vi "Main Chroma 19053 hipot.vi"   [LabVIEW 2018]
types:
  T1 = cluster{"error":bool, "code":i8, "source":string}
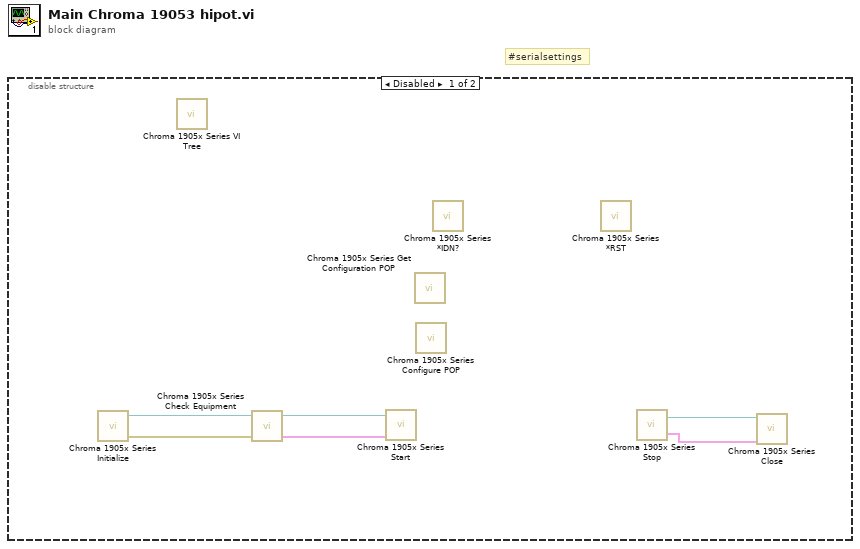
[diagram p0: block diagram]
diagram:
  # "#serialsettings"
  n1 = disable-structure shown="Disabled" {
    frame Disabled {
      n2 = call "Chroma 1905x Series Initialize.vi"() -> ("error out"=w5:errorcluster, "VISA session"=w6:refnum<visa-resource-name>)  [unwired: 4 in, 1 out]
      n3 = call "Chroma 1905x Series VI Tree.vi"() -> ()  [unwired: 1 in]
      n4 = call "Chroma 1905x Series Check Equipment.vi"("inst handle in"=w6, "error in"=w5) -> ("inst handle out"=w4:refnum<visa-resource-name>, "error out"=w3:T1)  [unwired: 5 in, 1 out]
      n5 = call "Chroma 1905x Series Start.vi"("inst handle in"=w4, "error in"=w3) -> ()  [unwired: 6 in, 2 out]
      n6 = call "Chroma 1905x Series Get Configuration POP.vi"() -> ()  [unwired: 7 in, 2 out]
      n7 = call "Chroma 1905x Series Configure POP.vi"() -> ()  [unwired: 25 in, 3 out]
      n8 = call "Chroma 1905x Series *IDN?.vi"() -> ()  [unwired: 3 in, 3 out]
      n9 = call "Chroma 1905x Series *RST.vi"() -> ()  [unwired: 4 in, 2 out]
      n10 = call "Chroma 1905x Series Stop.vi"() -> ("error out"=w2:T1, "inst handle out"=w1:refnum<visa-resource-name>)  [unwired: 3 in]
      n11 = call "Chroma 1905x Series Close.VI"("error in (no error)"=w2, "VISA session"=w1) -> ()  [unwired: 2 in, 1 out]
    }
    frame Enabled {
    }
  }
